vi "Read MQTTVersion.vi"(11 "ControlPacket in":refnum<class "ControlPacket.lvclass">) -> (2 "MQTTVersion":refnum<class "MQTTVersion.lvclass">, 3 "ControlPacket out":refnum<class "ControlPacket.lvclass">)   [LabVIEW 2013, in "MQTT_Control_Packets.lvlib" / "ControlPacket.lvclass"]
uses:
  ControlPacket.lvclass
  MQTT_311/MQTTVersion.lvclass
  ControlPacket.lvclass/ControlPacket.ctl
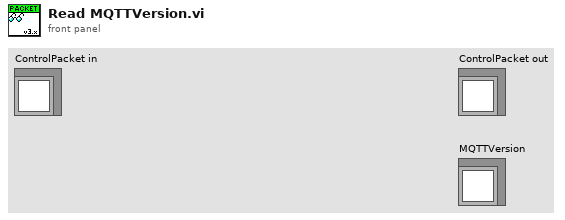
[diagram p1: front panel]
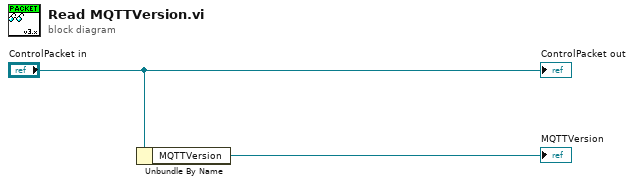
[diagram p0: block diagram]
diagram:
  n1 = Unbundle By Name("ControlPacket in") -> ("MQTTVersion"=→"MQTTVersion":refnum<class "MQTTVersion.lvclass">)
  "ControlPacket out" <- "ControlPacket in"
